vi "Set New Status.vi"(8 "error in (no error)":errorcluster, 10 "Status":T1, 11 "abs_Parallel in":refnum<class "bt_Parallel.lvclass">) -> (0 "error out":errorcluster, 3 "abs_Parallel out":refnum<class "bt_Parallel.lvclass">)   [LabVIEW 2021, in "BT.lvlib" / "bt_Parallel.lvclass"]
uses:
  bt_Parallel.lvclass
  C:/Users/Tim/Documents/GitHub/LV_Behaviour_Tree/Source/Support/Nodes/Composites/abs_Composite/bt_Composite.lvclass
  abs_Node/Status.ctl
  abs_Composite/bt_Composite.lvclass/bt_Composite.ctl
  bt_Parallel.lvclass/bt_Parallel.ctl
  abs_Composite/Properties/Read Index.vi
  abs_Node/bt_Node.lvclass
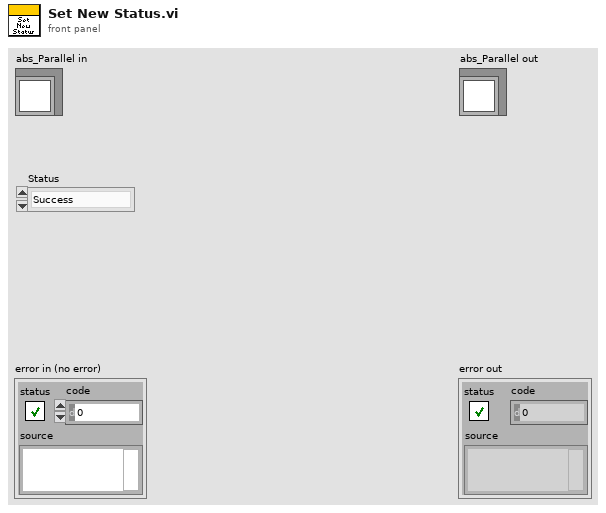
[diagram p1: front panel]
types:
  T1 = typedef "BT.lvlib/bt_Node.lvclass/Status.ctl" = enum16{"Success", "Failure", "Running"}
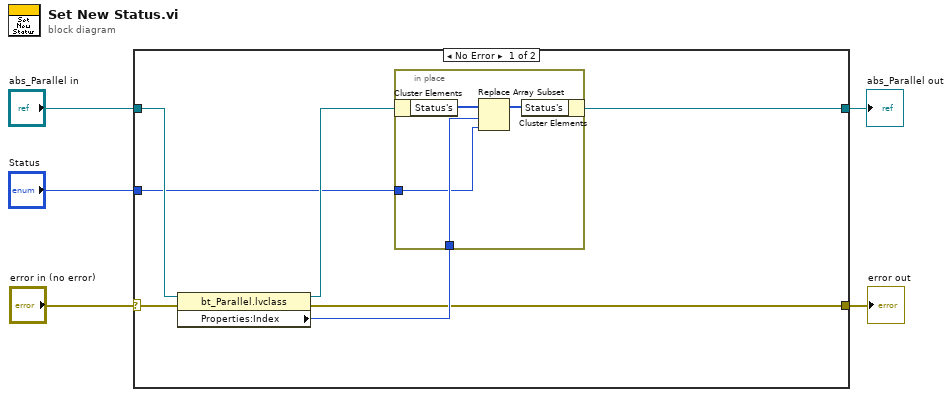
[diagram p0: block diagram]
diagram:
  n1 = case shown="No Error" "error in (no error)" {
    selector: "error in (no error)" -> [w12 w18]
    tunnel: [w7 w18] -> w4
    tunnel: [w8 w17] -> w2
    tunnel: "abs_Parallel in" -> [w11 w17]
    tunnel: "Status" -> [w6 _]
    frame No Error {
      n2 = property class="bt_Parallel.lvclass"(reference=w11, error in=w12) -> (reference out=w10:refnum<class "bt_Parallel.lvclass">, error out=w7:errorcluster, "Properties:Index"=w9:i32)
      n3 = in-place {
        in-place-border: w9 -> [w15]
        in-place-border: w6 -> [w13]
        n4 = in-place-cluster #1(w10) -> ("Status's"=w16:T1[])
        n5 = Replace Array Subset(array=w16, new element=w13, index=w15) -> (w14:T1[])
        n6 = in-place-cluster #1("Status's"=w14) -> (w8:refnum<class "bt_Parallel.lvclass">)
      }
    }
    frame Error {
    }
  }
  "error out" <- w4
  "abs_Parallel out" <- w2
